vi "mbug_2820_cont_acq.vi"() -> ()   [LabVIEW 2014]
doc: "This example shows how to acquire a power measurement using the VIs of the driver."
uses:
  <vilib>/Platform/TimedLoop/XDataNode/timing_clust.ctl
  <vilib>/Platform/TimedLoop/XDataNode/nitl_modes.ctl
  <vilib>/Platform/TimedLoop/XDataNode/wakeup.ctl
  <instrlib>/MBUG-2820/Private/Open_serial.vi
  <vilib>/platform/TimedLoop/XDataNode/XDataNode.xnode
  <instrlib>/MBUG-2820/MBUG-2820.lvlib
  <vilib>/Platform/TimedLoop/XDataNode/XDNodeRunTimeDep.lvlib
panel:
  out "Acq. points":u32
  out "Humidity graph":cluster{"X":dbl[], "Y":dbl[]}[](graph)
  out "Acq. time (sec)":dbl format="%.2f"
  out "Temperature graph":cluster{"X":dbl[], "Y":dbl[]}[](graph)
  in  "Stop acquisition":bool
  in  "Meas. interval (sec)":dbl=0.2 min=0.2 step=0.2
  out "Rel. humidity (%)":dbl format="%.2f"
  in  "Device serial (0: any)":u32 max=999999
  out "Temperature (°C)":dbl format="%#.3f"
  # "MBUG-2820 continuous acquisition example"
  # "Choose a device serial to open. ( 0: open the first available device.)"
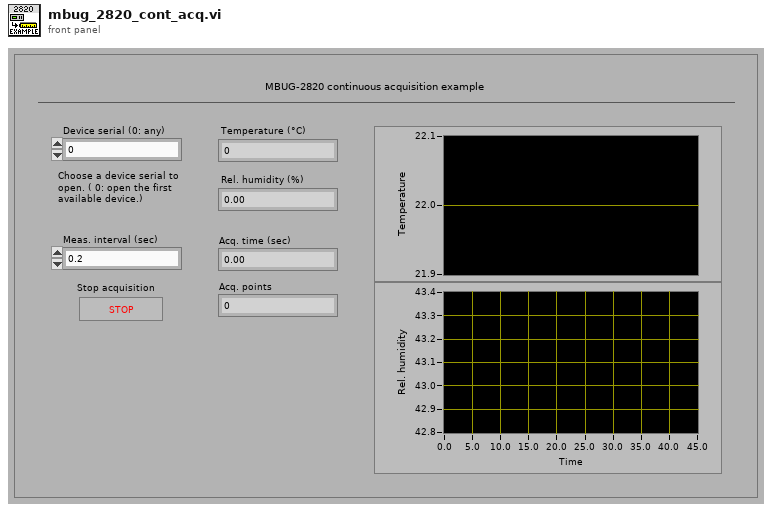
[diagram p1: front panel]
types:
  T1 = typedef "XDNodeRunTimeDep.lvlib/timing_clust.ctl" = cluster{"Expected End [f-1]":u64, "Actual End [f-1]":u64, "Finished Late? [f-1]":bool, "Expected End [i-1]":u64, "Actual End [i-1]":u64, "Finished Late? [i-1]":bool, "Expected Start [i]":u64, "Actual Start [i]":u64, "Expected Start [f]":u64, "Actual Start [f]":u64, "Source Name":string, "Structure Name":string, "Period":i64, "Deadline":i64, "Offset":i64, "Start":i64, "Priority":i32, "Timeout":i32, "Mode":T2, "Wakeup Reason":T3, "Error":errorcluster, "Source Type":string, "Secondary Source Type":string, "Global End Time":u64, "Global Start Time":u64, "Frame Duration":u64, "Iteration Duration":u64, "Assigned CPU":i32, "I/O Scan Engine Mode":u32}
  T2 = typedef "XDNodeRunTimeDep.lvlib/nitl_modes.ctl" = enum32{"No Change", "Process missed periods, maintain original phase", "Discard missed periods, maintain original phase", "Process missed periods, ignore original phase", "Discard missed periods, ignore original phase"}
  T3 = typedef "XDNodeRunTimeDep.lvlib/wakeup.ctl" = enum32{"Normal", "Aborted", "Asynchronous wakeup", "Timing source error", "Timed loop error", "Timeout"}
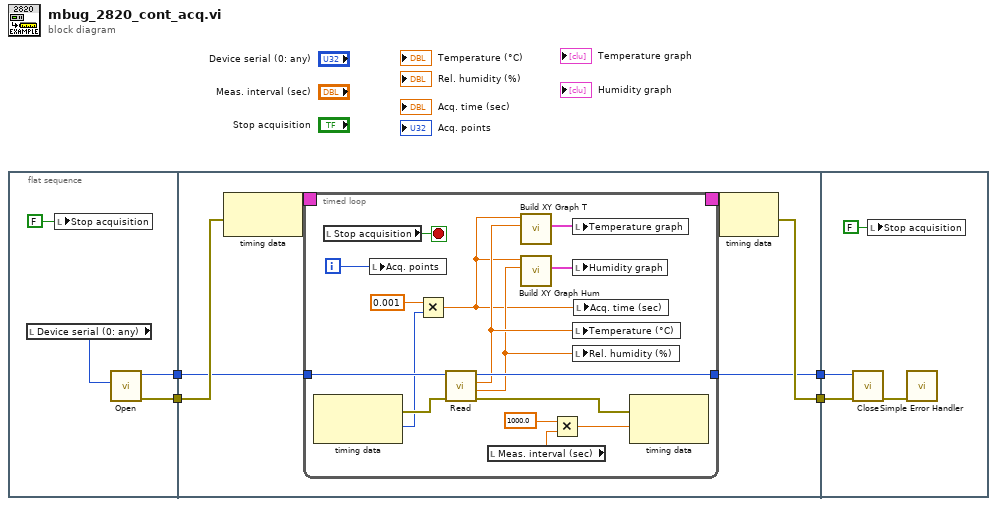
[diagram p0: block diagram]
diagram:
  n1 = flat-sequence {
    tunnel: [w8] -> w4
    tunnel: [w7] -> w3
    tunnel: w4 -> [w12]
    tunnel: w3 -> [w11]
    tunnel: [w10] -> w2
    tunnel: [w9] -> w1
    tunnel: w2 -> [w45]
    tunnel: w1 -> [w44]
    frame #0 {
      n2 = local read "Device serial (0: any)"() -> (w5:u32)
      n3 = local write "Stop acquisition"(FALSE ("Stop acquisition")) -> ()
      n4 = call-poly <instrlib>:"Open.vi"("Device serial (0=any)"=w5) -> ("error out"=w8:errorcluster, "Device handle"=w7:u32)  [unwired: 5 in]
    }
    frame #1 {
      n5 = node-c288(w12) -> (w14:T1)
      n6 = timed-loop {
        timing: w14 -> [_]
        timing-out: [_] -> w13
        tunnel: w11 -> [w30]
        tunnel: [w28] -> w9
        i -> [w25]
        stop <- w24 stop-if-true
        n7 = node-c288() -> (w29:errorcluster, w19:i64)  [unwired: 1 in]
        n8 = local read "Stop acquisition"() -> (w24:bool)
        n9 = local write "Acq. points"(w25) -> ()
        n10 = Multiply(x=0.001 ("y"), y=w19) -> (x*y=w17:dbl)
        n11 = call <instrlib>:"Read.vi"("error in (no error)"=w29, "Device handle in"=w30) -> ("error out"=w27:errorcluster, "Rel. humidity (%)"=w20:dbl, "Temperature (°C)"=w21:dbl, "Device handle out"=w28:u32)  [unwired: 2 in]
        n12 = local read "Meas. interval (sec)"() -> (w15:dbl)
        n13 = call "Build XY Graph T"("Y Input"=w21, "X Input"=w17) -> ("XY Graph"=w23:cluster{"X":dbl[], "Y":dbl[]}[])  [unwired: 8 in, 1 out]
        n14 = call "Build XY Graph Hum"("Y Input"=w20, "X Input"=w17) -> ("XY Graph"=w22:cluster{"X":dbl[], "Y":dbl[]}[])  [unwired: 8 in, 1 out]
        n15 = Multiply(x=1000.0 ("y"), y=w15) -> (x*y=w26:dbl)
        n16 = local write "Temperature graph"(w23) -> ()
        n17 = local write "Humidity graph"(w22) -> ()
        n18 = local write "Temperature (°C)"(w21) -> ()
        n19 = local write "Rel. humidity (%)"(w20) -> ()
        n20 = local write "Acq. time (sec)"(w17) -> ()
        n21 = node-c288(w27, w26) -> ()  [unwired: 1 out]
      }
      n22 = node-c288(w13) -> (w10:errorcluster)
    }
    frame #2 {
      n23 = call <instrlib>:"Close.vi"("error in (no error)"=w45, "Device handle"=w44) -> ("error out"=w46:errorcluster)  [unwired: 5 in]
      n24 = local write "Stop acquisition"(FALSE ("Stop acquisition")) -> ()
      n25 = call <vilib>:"Simple Error Handler.vi"("error in (no error)"=w46) -> ()  [unwired: 4 in, 5 out]
    }
  }
